vi "HWT_Shared_Proc_Globals.vi"() -> ()   [LabVIEW 2015]
panel:
  out "Exe?":bool
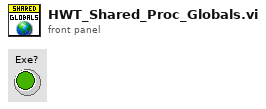
[diagram p1: front panel]
diagram:
